vi "Update.vi"(6 "Table Name":string, 7 "condition":string, 8 "error in (no error)":errorcluster, 9 "Data List":string, 10 "ColumnName List":string, 11 "MySQL in":refnum<class "MySQL.lvclass">) -> (0 "error out":errorcluster, 2 "SQL Query":string, 3 "MySQL out":refnum<class "MySQL.lvclass">)   [LabVIEW 2021]
uses:
  MySQL.lvclass
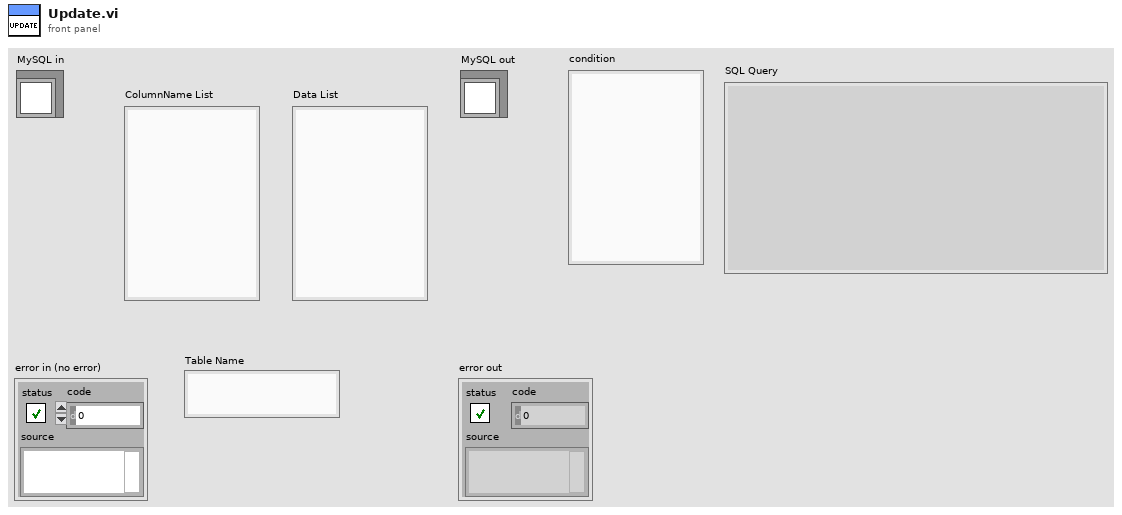
[diagram p1: front panel]
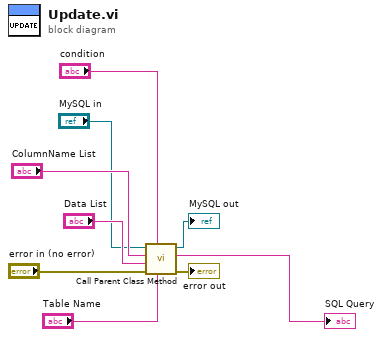
[diagram p0: block diagram]
diagram:
  n1 = call-parent "Call Parent Class Method"("Table Name"="Table Name", "condition"="condition", "error in (no error)"="error in (no error)", "Data List"="Data List", "ColumnName List"="ColumnName List", "DataBase_SQL in"="MySQL in") -> ("error out"=→"error out":errorcluster, "SQL Query"=→"SQL Query":string, "DataBase_SQL out"=→"MySQL out":refnum<class "MySQL.lvclass">)  [unwired: 3 in]
